vi "Graphics-Convert dotNET Rect.vi"(1 ".NET Refnum in":refnum<k24>) -> (0 "Rect":T1)   [LabVIEW 2015]
uses:
  Rectangle (double).ctl
  System.Drawing
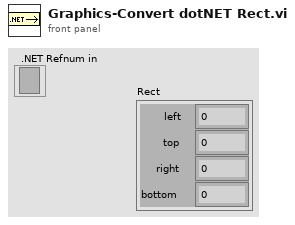
[diagram p1: front panel]
types:
  T1 = typedef "Rectangle (double).ctl" = cluster{"left":dbl, "top":dbl, "right":dbl, "bottom":dbl}
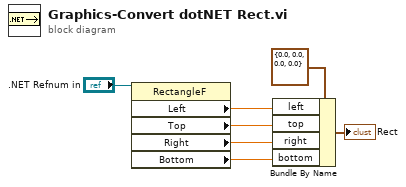
[diagram p0: block diagram]
diagram:
  n1 = property class="RectangleF"(reference=".NET Refnum in") -> ("Left"=w2:sgl, "Top"=w3:sgl, "Right"=w5:sgl, "Bottom"=w6:sgl)  [unwired: 1 in, 2 out]
  n2 = Bundle By Name(cluster=T1 {"left"=0.0, "top"=0.0, "right"=0.0, "bottom"=0.0} ("rect"), "left"=w2, "top"=w3, "right"=w5, "bottom"=w6) -> (→"Rect":T1)
